vi "Set Pressure.vi"(8 "error in (no error)":errorcluster, 10 "Pressure (bar)":dbl, 11 "Cylinder in":refnum<class "Cylinder.lvclass">) -> (0 "error out":errorcluster, 3 "Cylinder out":refnum<class "Cylinder.lvclass">)   [LabVIEW 2015, in "cRIO-Carbondioxide.lvlib" / "CO2-Actor.lvlib" / "Cylinder.lvclass"]
uses:
  Cylinder.lvclass
  Cylinder.lvclass/Cylinder.ctl
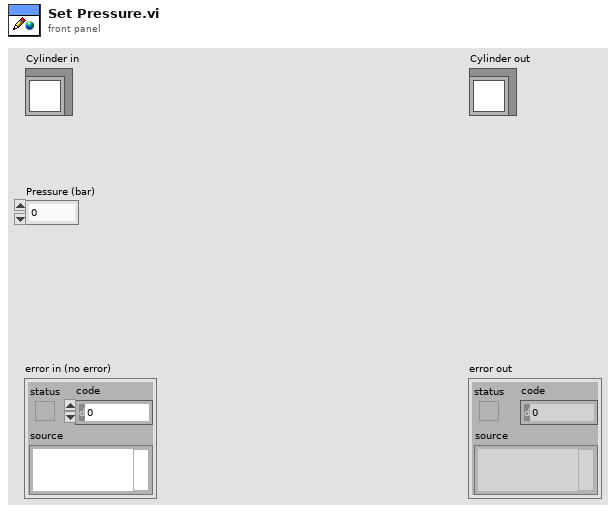
[diagram p1: front panel]
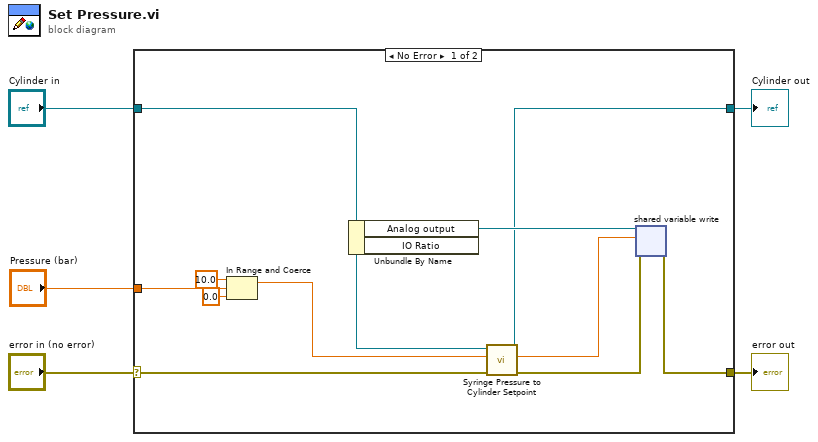
[diagram p0: block diagram]
diagram:
  n1 = case shown="No Error" "error in (no error)" {
    selector: "error in (no error)" -> [w11 w18]
    tunnel: [w15 w18] -> w4
    tunnel: [w7 w17] -> w2
    tunnel: "Cylinder in" -> [w8 w17]
    tunnel: "Pressure (bar)" -> [w14 _]
    frame No Error {
      n2 = In Range and Coerce(upper limit=10.0, x=w14, lower limit=0.0) -> (coerced(x)=w9:dbl)  [unwired: 1 out]
      n3 = Unbundle By Name(w8) -> ("Analog output"=w16:refnum<k21>)  [unwired: 1 out]
      n4 = call "Syringe Pressure to Cylinder Setpoint.vi"("error in (no error)"=w11, "Syringe Pressure"=w9, "Cylinder in"=w8) -> ("error out"=w10:errorcluster, "Cylinder Setpoint"=w6:dbl, "Cylinder out"=w7:refnum<class "Cylinder.lvclass">)  [unwired: 6 in]
      n5 = shared-variable-write(w16, w10, w6) -> (w15:errorcluster)  [unwired: 1 out]
    }
    frame Error {
    }
  }
  "error out" <- w4
  "Cylinder out" <- w2
